vi "Init UI.vi"(6 "error in (no error)":errorcluster, 8 "User Iterface Data":T1, 9 "MHL References":T3) -> (0 "error out":errorcluster, 2 "User Iterface Data out":T1, 3 "MHL Data":T4)   [LabVIEW 2024]
uses:
  MHL Data.ctl
  User Interface Data.ctl
  Controls/Car Wash Indicators.ctl
  MHL References.ctl
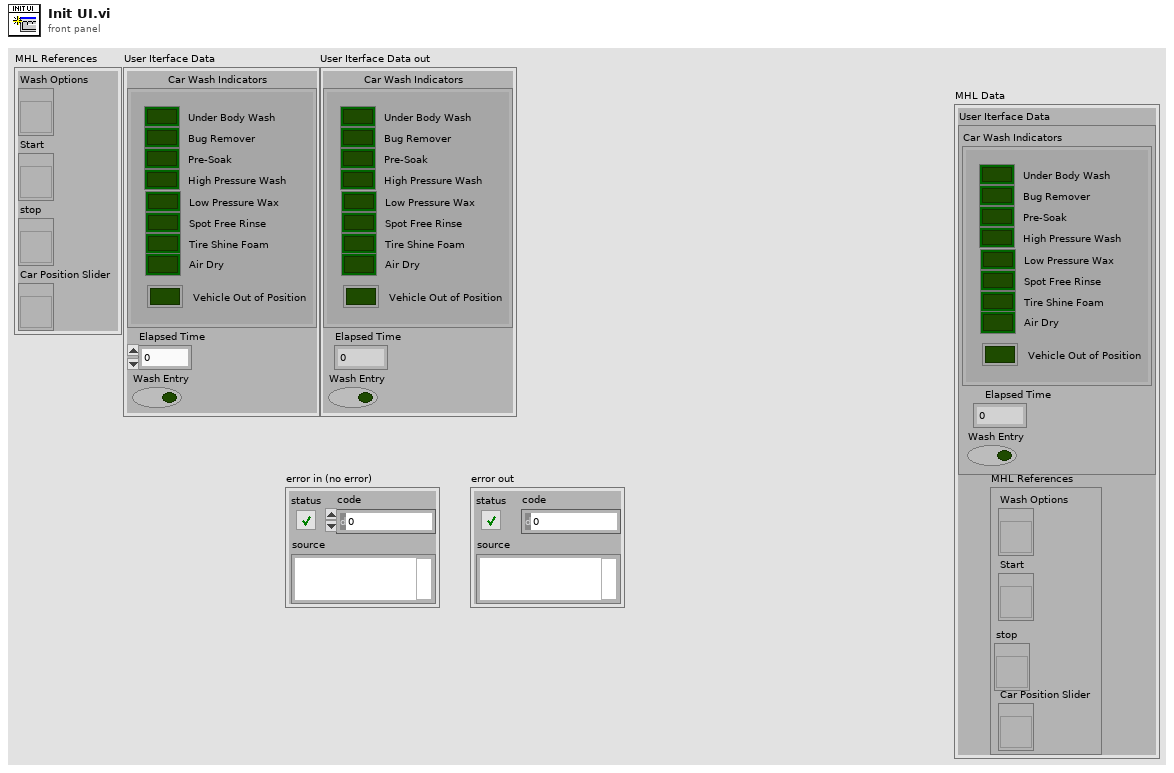
[diagram p1: front panel]
types:
  T1 = typedef "User Interface Data.ctl" = cluster{"Car Wash Indicators":T2, "Elapsed Time":dbl, "Wash Entry":bool}
  T2 = typedef "Car Wash Indicators.ctl" = cluster{"Under Body Wash":bool, "Bug Remover":bool, "Pre-Soak":bool, "High Pressure Wash":bool, "Low Pressure Wax":bool, "Spot Free Rinse":bool, "Tire Shine Foam":bool, "Air Dry":bool, "Vehicle Out of Position":bool}
  T3 = typedef "MHL References.ctl" = cluster{"Wash Options":refnum<vi>, "Start":refnum<vi>, "stop":refnum<vi>, "Car Position Slider":refnum<vi>}
  T4 = typedef "MHL Data.ctl" = cluster{"User Iterface Data":T1, "MHL References":T3}
  T5 = cluster{"[0]":bool, "[1]":bool, "[2]":bool, "[3]":bool, "[4]":bool, "[5]":bool, "[6]":bool, "[7]":bool, "[8]":bool}
  T6 = enum8{"Enabled", "Disabled", "Disabled and Grayed Out"}
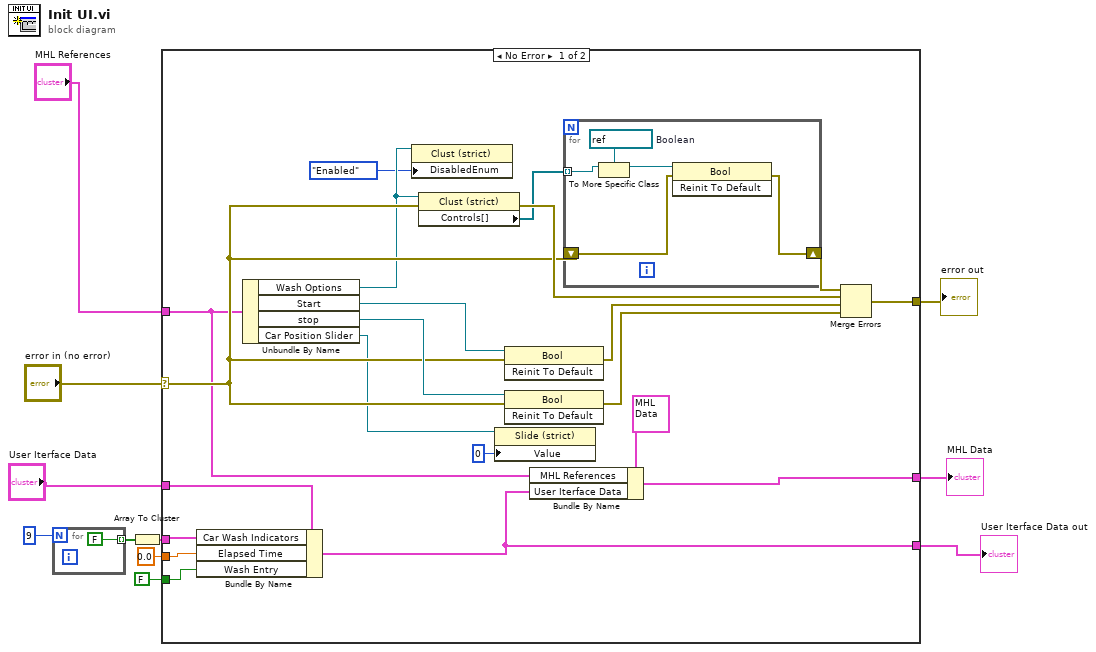
[diagram p0: block diagram]
diagram:
  n1 = for {
    N: 9 -> [_]
    tunnel: [FALSE] -> w8 mode=indexing
  }
  n2 = Array To Cluster(array=w8) -> (cluster=w7:T5)
  n3 = case shown="No Error" "error in (no error)" {
    selector: "error in (no error)" -> [w26 w39]
    tunnel: [w33 w39] -> w11
    tunnel: "MHL References" -> [w18 _]
    tunnel: "User Iterface Data" -> [w24 _]
    tunnel: w7 -> [w23 _]
    tunnel: 0.0 ("Elapsed Time") -> [w22 _]
    tunnel: FALSE ("Wash Entry") -> [w21 _]
    tunnel: [w20 _] -> w1
    tunnel: [w17 _] -> w4
    frame No Error {
      n4 = Bundle By Name(cluster=w24, "Car Wash Indicators"=w23, "Elapsed Time"=w22, "Wash Entry"=w21) -> (w20:T1)
      n5 = Unbundle By Name(w18) -> ("Wash Options"=w16:refnum<vi>, "Start"=w28:refnum<vi>, "stop"=w29:refnum<vi>, "Car Position Slider"=w14:refnum<vi>)
      n6 = property class="Clust (strict)"(reference=w16, "DisabledEnum"=T6."Enabled" ("Disabled")) -> ()  [unwired: 1 in, 2 out]
      n7 = property class="Clust (strict)"(reference=w16, error in=w26) -> (error out=w30:errorcluster, "Controls[]"=w27:refnum<vi>[])  [unwired: 1 out]
      n8 = property class="Slide (strict)"(reference=w14, "Value"=u8 0) -> ()  [unwired: 1 in, 2 out]
      n9 = invoke class="Bool" method="Reinit To Default"(reference=w28, error in=w26) -> (error out=w31:errorcluster)  [unwired: 1 in, 2 out]
      n10 = invoke class="Bool" method="Reinit To Default"(reference=w29, error in=w26) -> (error out=w25:errorcluster)  [unwired: 1 in, 2 out]
      n11 = Bundle By Name(cluster=T4 {"User Iterface Data"={"Car Wash Indicators"={"Under Body Wash"=FALSE, "Bug Remover"=FALSE, "Pre-Soak"=FALSE, "High Pressure Wash"=FALSE, "Low Pressure Wax"=FALSE, "Spot Free Rinse"=FALSE, "Tire Shine Foam"=FALSE, "Air Dry"=FALSE, "Vehicle Out of Position"=FALSE}, "Elapsed Time"=0.0, "Wash Entry"=FALSE}, "MHL References"={"Wash Options"=refnum, "Start"=refnum, "stop"=refnum, "Car Position Slider"=refnum}} ("MHL Data"), "MHL References"=w18, "User Iterface Data"=w20) -> (w17:T4)
      n12 = for {
        tunnel: w27 -> [w38] mode=indexing
        shift-right: [w34] -> w32
        shift-left: w26 -> [w35]
        w37 = refnum<vi> refnum  # Boolean
        n13 = To More Specific Class(target class=w37, reference=w38) -> (specific class reference=w36:refnum<vi>)  [unwired: 1 in, 1 out]
        n14 = invoke class="Bool" method="Reinit To Default"(reference=w36, error in=w35) -> (error out=w34:errorcluster)  [unwired: 1 in, 2 out]
      }
      n15 = Merge Errors(w30, w31, w25, w32) -> (w33:errorcluster)
    }
    frame Error {
    }
  }
  "error out" <- w11
  "MHL Data" <- w4
  "User Iterface Data out" <- w1
